vi "ScaraInverseKinematics.vi"(4 "Y0":dbl, 5 "X0":dbl, 6 "L3":dbl, 8 "L2":dbl, 9 "L1":dbl, 10 "Y":dbl, 11 "X":dbl) -> (2 "angle 2":dbl, 3 "angle 1":dbl)   [LabVIEW 2014]
doc: "Using the length of the arms L1, L2, and L3, calculates the angles angle 1 and angle 2 of the 2 arms of a Scara Robot. Positive a2? is a boolean that selects the positive value of angle 2 as a solution if true."
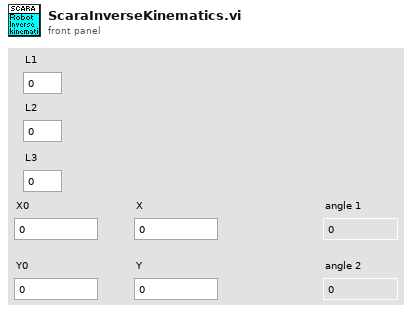
[diagram p1: front panel]
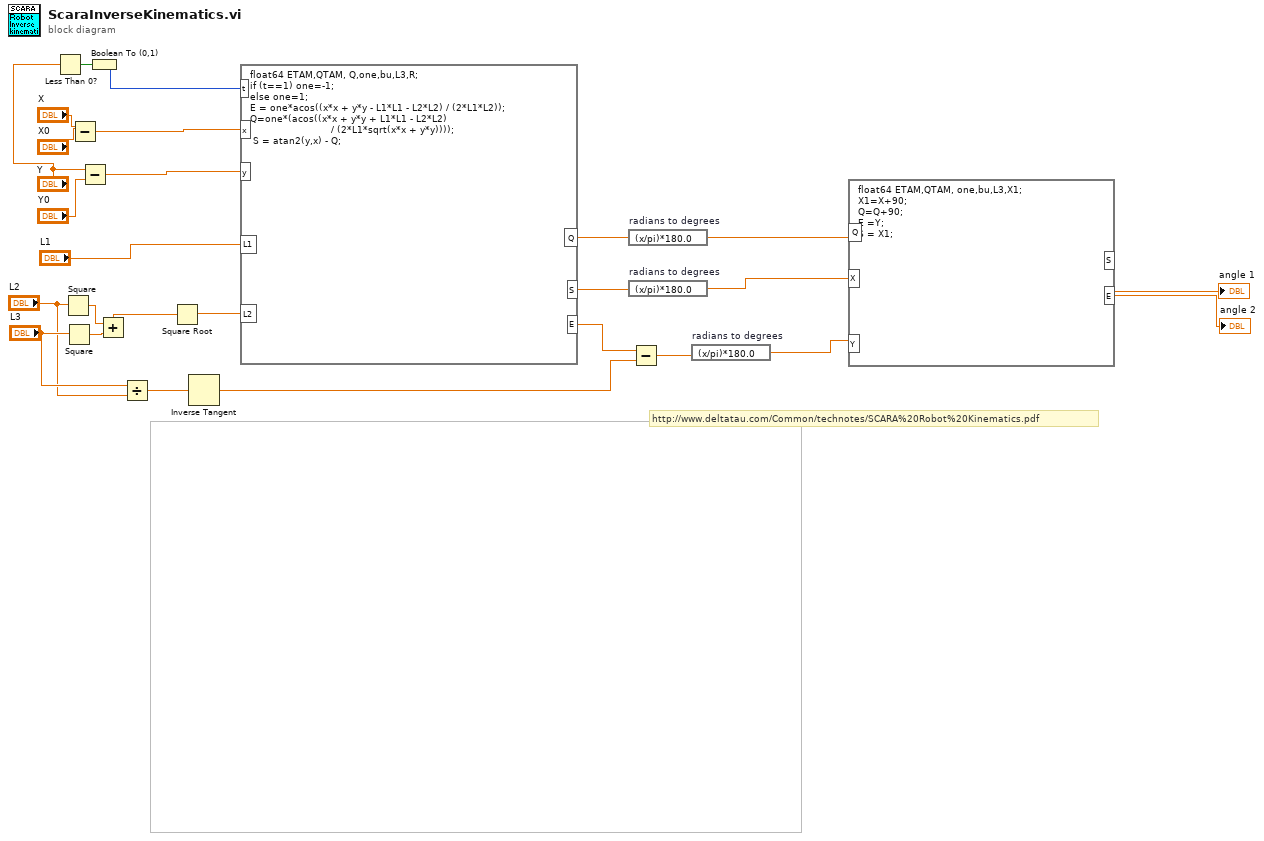
[diagram p0: block diagram]
diagram:
  # "http://www.deltatau.com/Common/technotes/SCARA%20Robot%20Kinematics.pdf"
  n1 = Less Than 0?(x="Y") -> (x < 0?=w1:bool)
  n2 = Square(x="L2") -> (x^2=w21:dbl)
  n3 = Square(x="L3") -> (x^2=w25:dbl)
  n4 = Subtract(x="X", y="X0") -> (x-y=w12:dbl)
  n5 = Subtract(x="Y", y="Y0") -> (x-y=w13:dbl)
  n6 = Boolean To (0,1)(Boolean=w1) -> (0, 1=w14:i16)
  n7 = Add(x=w21, y=w25) -> (x+y=w24:dbl)
  n8 = Divide(x="L3", y="L2") -> (x/y=w20:dbl)
  n9 = Square Root(x=w24) -> (sqrt(x)=w23:dbl)
  n10 = Inverse Tangent(1:w20) -> (0:w18:dbl)
  n11 = formula code="float64 ETAM,QTAM, Q,one,bu,L3,R;\nif (t==1) one=-1;\nelse one=1;\nE = one*acos((x*x + y*y - L1*L1 - L2*L2) / (2*L1*L2));\nQ=one*(acos((x*x + y*y + L1*L1 - L2*L2)\n                           / (2*L1*sqrt(x*x + y*y))));\n S = atan2(y,x) - Q;"("x"=w12, "y"=w13, "L1"="L1", "L2"=w23, "t"=w14) -> ("E"=w19:dbl, "S"=w17:dbl, "Q"=w4:dbl)
  n12 = expression code="(x/pi)*180.0" "radians to degrees"(w4) -> (w3:dbl)
  n13 = expression code="(x/pi)*180.0" "radians to degrees"(w17) -> (w8:dbl)
  n14 = Subtract(x=w19, y=w18) -> (x-y=w16:dbl)
  n15 = expression code="(x/pi)*180.0" "radians to degrees"(w16) -> (w7:dbl)
  n16 = formula code="float64 ETAM,QTAM, one,bu,L3,X1;\nX1=X+90;\nQ=Q+90;\nE =Y;\nS = X1;"("X"=w8, "Y"=w7, "Q"=w3) -> ("E"=→"angle 2":dbl, "S"=→"angle 1":dbl)
